vi "16-ParseSubpacketsByBITS.vi"(10 "Number of BITS":u32, 11 "BITS in":bool[](array[boolean])) -> (2 "Sub Packets":T1(array[cluster]), 3 "BITS out":bool[](array[boolean]))   [LabVIEW 2019, in "16.lvlib"]
uses:
  16.lvlib
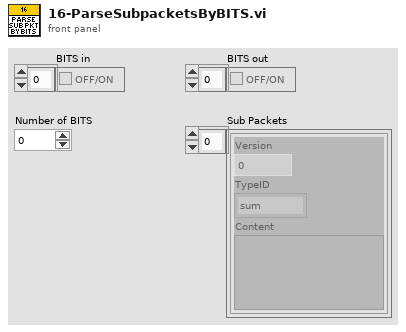
[diagram p1: front panel]
types:
  T1 = cluster{"Version":u32, "TypeID":enum16{"sum", "product", "minimum", "maximum", "literal", "greater than", "less than", "equal to"}, "Content":variant}[]
  T2 = cluster{"Version":u32, "TypeID":enum16{"sum", "product", "minimum", "maximum", "literal", "greater than", "less than", "equal to"}, "Content":variant}
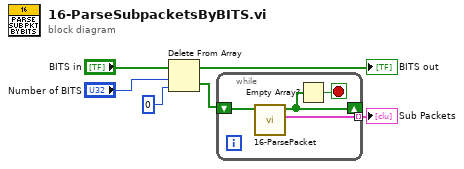
[diagram p0: block diagram]
diagram:
  n1 = Delete From Array(array="BITS in", length="Number of BITS", index=0) -> (deleted portion=w6:bool[], array with subset deleted=→"BITS out":bool[])
  n2 = while {
    tunnel: [w10] -> w4 mode=indexing
    shift-right: [w8] -> _
    shift-left: w6 -> [w9]
    stop <- w7 stop-if-true
    n3 = call "16-ParsePacket.vi"("BITS in"=w9) -> ("Packet"=w10:T2, "BITS out"=w8:bool[])  [unwired: 9 in]
    n4 = Empty Array?(array=w8) -> (empty?=w7:bool)
  }
  "Sub Packets" <- w4
